vi "Authorization.vi"() -> (3 "SetAuthorizationCode":bool)   [LabVIEW 2020, in "HslCommunication.lvlib"]
uses:
  HslCommunication.lvlib
  D:/Git/Labview-Libraries/Libraries/HslCommunication/_Dependenciecs/HslCommunication.dll
  _Dependenciecs/HslCommunication.dll
panel:
  out "error out":errorcluster
  in  "error in (no error)":errorcluster
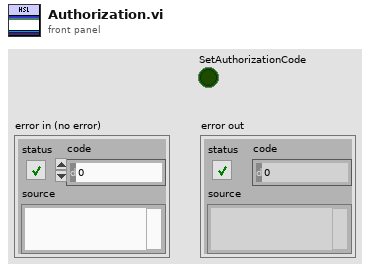
[diagram p1: front panel]
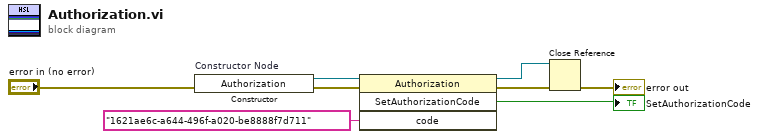
[diagram p0: block diagram]
diagram:
  n1 = constructor on="Constructor Node" class="Authorization"(error in="error in (no error)") -> (reference out=w8:refnum<k24>, error out=w4:errorcluster)  [unwired: 2 in, 1 out]
  n2 = invoke class="Authorization" method="SetAuthorizationCode"(reference=w8, error in=w4, "code"="1621ae6c-a644-496f-a020-be8888f7d711") -> (reference out=w6:refnum<k24>, error out=w7:errorcluster, "SetAuthorizationCode"=→"SetAuthorizationCode":bool)  [unwired: 1 in, 1 out]
  n3 = Close Reference(reference=w6, error in (no error)=w7) -> (error out=→"error out":errorcluster)
